vi "Get TestStand Notifier Info.vi"(8 "error in (no error)":errorcluster, 10 "Notifier":string="TemperatureNotifier", 11 "SequenceContext":refnum<k7>) -> (0 "error out":errorcluster, 3 "Stop":bool)   [LabVIEW 2025]
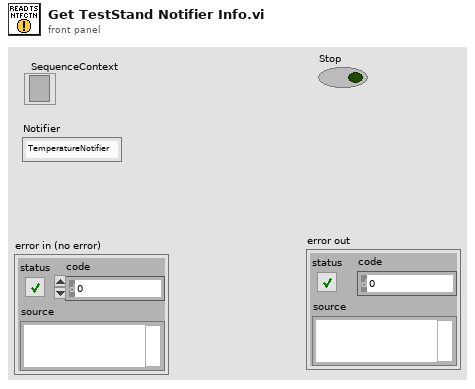
[diagram p1: front panel]
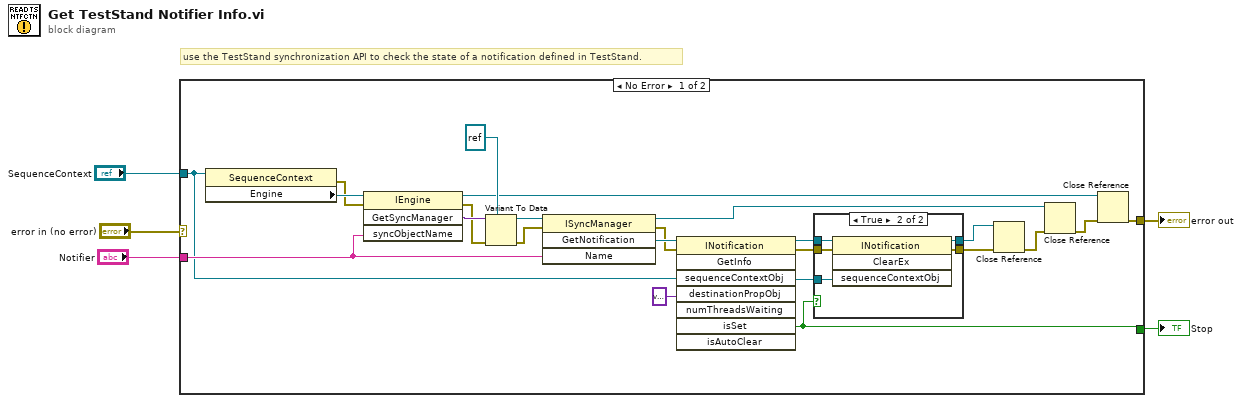
[diagram p0: block diagram]
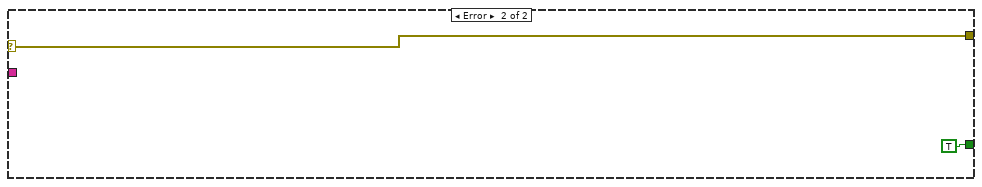
[diagram p3: hidden frame]
diagram:
  # "use the TestStand synchronization API to check the state of a notification defined in TestStand."
  n1 = case shown="No Error" "error in (no error)" {
    selector: "error in (no error)" -> [_ w35]
    tunnel: [w6 TRUE ("isSet")] -> w5
    tunnel: "SequenceContext" -> [w9 _]
    tunnel: [w13 w35] -> w3
    tunnel: "Notifier" -> [w12 _]
    frame No Error {
      n2 = property class="SequenceContext"(reference=w9) -> (error out=w18:errorcluster, "Engine"=w23:refnum<k7>)  [unwired: 1 in, 1 out]
      n3 = invoke class="IEngine" method="GetSyncManager"(reference=w23, error in=w18, "syncObjectName"=w12) -> (reference out=w20:refnum<k7>, error out=w17:errorcluster, "GetSyncManager"=w24:variant)  [unwired: 1 in, 1 out]
      n4 = Variant To Data(error in=w17, type=refnum<k7> refnum ("reference out"), Variant=w24) -> (data=w26:refnum<k7>, error out=w16:errorcluster)
      n5 = invoke class="ISyncManager" method="GetNotification"(reference=w26, error in=w16, "Name"=w12) -> (reference out=w21:refnum<k7>, error out=w15:errorcluster, "GetNotification"=w27:refnum<k7>)  [unwired: 1 in, 1 out]
      n6 = invoke class="INotification" method="GetInfo"(reference=w27, error in=w15, "sequenceContextObj"=w9, "destinationPropObj"=variant) -> (reference out=w11:refnum<k7>, error out=w10:errorcluster, "isSet"=w6:bool)  [unwired: 4 in, 5 out]
      n7 = case shown="True" w6 {
        tunnel: w11 -> [w28 w34]
        tunnel: w10 -> [w29 w33]
        tunnel: w9 -> [_ w32]
        tunnel: [w29 w31] -> w8
        tunnel: [w28 w30] -> w7
        frame False {
        }
        frame True {
          n8 = invoke class="INotification" method="ClearEx"(reference=w34, error in=w33, "sequenceContextObj"=w32) -> (reference out=w30:refnum<k7>, error out=w31:errorcluster)  [unwired: 1 in, 2 out]
        }
      }
      n9 = Close Reference(reference=w7, error in (no error)=w8) -> (error out=w22:errorcluster)
      n10 = Close Reference(reference=w21, error in (no error)=w22) -> (error out=w19:errorcluster)
      n11 = Close Reference(reference=w20, error in (no error)=w19) -> (error out=w13:errorcluster)
    }
    frame Error {
    }
  }
  "Stop" <- w5
  "error out" <- w3
